vi "dfd_MRateObj_Get Coef WordLen.vi"(11 "multirate filter in":T1={"mMRate_Structure"=enum."FIR", "mMRate_Mode"=0, "mMRate_Factor"=1, "mMRate_FIRParams"={"mMRate_FIR_H"=[], "mMRate_FIR_IsNyquist?"=FALSE, "mMRate_FIR_IsSymmetric?"=FALSE}, "mMRate_CICParams"={"mMRate_CIC_#Stage"=2, "mMRate_CIC_Lag"=1, "mMRate_CIC_Type"=enum."Lowpass"}, "mMRate_Order"=0, "mMRate_Version"="2.0", "mMRate_Comments"="", "mMRate_RationalFactor"={"mMRate_L"=-1, "mMRate_M"=-1}, "mMRate_Fs"=1.0, "mMRate_Quantized?"=FALSE, "mMRate_QFilterGain"=1.0, "mMRate_CoefWl"=16, "mMRate_Scaling"={"mMRate_ScaleByPowerOf2?"=FALSE, "mMRate_ScaleType"=enum."Time Domain 1-Norm"}, "mMRate_InputWl"=16, "mMRate_OutputWl"=16, "mMRate_OutputMode"=enum."Nearest", "mMRate_MultMode"=enum."Truncated", "mMRate_BitPruning"=FALSE, "mMRate_GainWl"=16, "mMRate_OutputFwl"=0, "mMRate_SumIwl"=0, "mMRate_InputIwl "=16, "mMRate_SumWl"=32, "mMRate_CoefIwl"=0} {"mMRate_SumWl" min=1 max=32 step=1; "mMRate_InputIwl" min=1 max=32 step=1; "mMRate_GainWl" min=1 max=32 step=1; "mMRate_OutputWl" min=1 max=32 step=1; "mMRate_InputWl" min=1 max=32 step=1; "mMRate_CoefWl" min=1 max=32 step=1; "mMRate_Mode" items=["Default"=-1, "No Rate Change"=0, "Interpolation"=1, "Decimation"=2, "Interpolated"=3, "Rational"=4]}) -> (2 "coef wl":i16, 3 "dup multirate filter":T1={"mMRate_Structure"=enum."FIR", "mMRate_Mode"=0, "mMRate_Factor"=1, "mMRate_FIRParams"={"mMRate_FIR_H"=[], "mMRate_FIR_IsNyquist?"=FALSE, "mMRate_FIR_IsSymmetric?"=FALSE}, "mMRate_CICParams"={"mMRate_CIC_#Stage"=2, "mMRate_CIC_Lag"=1, "mMRate_CIC_Type"=enum."Lowpass"}, "mMRate_Order"=0, "mMRate_Version"="2.0", "mMRate_Comments"="", "mMRate_RationalFactor"={"mMRate_L"=-1, "mMRate_M"=-1}, "mMRate_Fs"=1.0, "mMRate_Quantized?"=FALSE, "mMRate_QFilterGain"=1.0, "mMRate_CoefWl"=16, "mMRate_Scaling"={"mMRate_ScaleByPowerOf2?"=FALSE, "mMRate_ScaleType"=enum."Time Domain 1-Norm"}, "mMRate_InputWl"=16, "mMRate_OutputWl"=16, "mMRate_OutputMode"=enum."Nearest", "mMRate_MultMode"=enum."Truncated", "mMRate_BitPruning"=FALSE, "mMRate_GainWl"=16, "mMRate_OutputFwl"=0, "mMRate_SumIwl"=0, "mMRate_InputIwl "=16, "mMRate_SumWl"=32, "mMRate_CoefIwl"=0} {"mMRate_SumWl" min=1 max=32 step=1; "mMRate_InputIwl" min=1 max=32 step=1; "mMRate_GainWl" min=1 max=32 step=1; "mMRate_OutputWl" min=1 max=32 step=1; "mMRate_InputWl" min=1 max=32 step=1; "mMRate_CoefWl" min=1 max=32 step=1; "mMRate_Mode" items=["Default"=-1, "No Rate Change"=0, "Interpolation"=1, "Decimation"=2, "Interpolated"=3, "Rational"=4]})   [LabVIEW 2017, in "NI_DigFilterLicensed.lvlib"]
uses:
  <vilib>/addons/Digital Filter Design/NI_DigFilterLicensed.lvlib
  <vilib>/addons/Digital Filter Design/_Objects.llb/DFD Multirate Filter Obj.ctl
  <vilib>/addons/Digital Filter Design/_Objects.llb/DFD Multirate Mode.ctl
  <vilib>/addons/Digital Filter Design/_Objects.llb/DFD Coef Norm Type.ctl
  <vilib>/addons/Digital Filter Design/_Objects.llb/DFD Round-off Mode.ctl
  <vilib>/addons/Digital Filter Design/_Objects.llb/DFD FXP MRate Multiply Mode.ctl
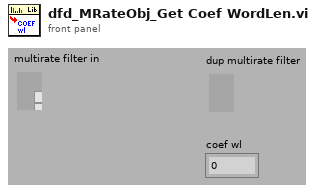
[diagram p1: front panel]
types:
  T1 = typedef "NI_DigFilterLicensed.lvlib/DFD Multirate Filter Obj.ctl" = cluster{"mMRate_Structure":enum16{"CIC", "FIR", "IIR", "Lattice"}, "mMRate_Mode":T2, "mMRate_Factor":i32, "mMRate_FIRParams":cluster{"mMRate_FIR_H":dbl[], "mMRate_FIR_IsNyquist?":bool, "mMRate_FIR_IsSymmetric?":bool}, "mMRate_CICParams":cluster{"mMRate_CIC_#Stage":i32, "mMRate_CIC_Lag":i32, "mMRate_CIC_Type":enum16{"Lowpass", "Highpass"}}, "mMRate_Order":i32, "mMRate_Version":string, "mMRate_Comments":string, "mMRate_RationalFactor":cluster{"mMRate_L":i32, "mMRate_M":i32}, "mMRate_Fs":dbl, "mMRate_Quantized?":bool, "mMRate_QFilterGain":dbl, "mMRate_CoefWl":i16, "mMRate_Scaling":cluster{"mMRate_ScaleByPowerOf2?":bool, "mMRate_ScaleType":T3}, "mMRate_InputWl":i16, "mMRate_OutputWl":i16, "mMRate_OutputMode":T4, "mMRate_MultMode":T5, "mMRate_BitPruning":bool, "mMRate_GainWl":i16, "mMRate_OutputFwl":i16, "mMRate_SumIwl":i16, "mMRate_InputIwl ":i16, "mMRate_SumWl":i16, "mMRate_CoefIwl":i16}
  T2 = typedef "NI_DigFilterLicensed.lvlib/DFD Multirate Mode.ctl" = i16
  T3 = typedef "NI_DigFilterLicensed.lvlib/DFD Coef Norm Type.ctl" = enum16{"No Norm", "Time Domain 1-Norm", "Time Domain 2-Norm", "Time Domain Inf-Norm"}
  T4 = typedef "NI_DigFilterLicensed.lvlib/DFD Round-off Mode.ctl" = enum16{"Nearest", "Truncation"}
  T5 = typedef "NI_DigFilterLicensed.lvlib/DFD FXP MRate Multiply Mode.ctl" = enum16{"Truncated", "Full"}
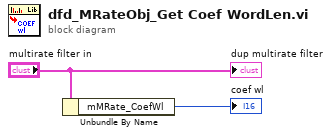
[diagram p0: block diagram]
diagram:
  n1 = Unbundle By Name("multirate filter in") -> ("mMRate_CoefWl"=→"coef wl":i16)
  "dup multirate filter" <- "multirate filter in"
